vi "Teleop.vi"(10 "Match Info":T1={"Autonomous Elapsed Seconds"=0.0, "TeleOp Elapsed Seconds"=0.0, "Disabled Elapsed Seconds"=0.0, "Visited Autonomous"=FALSE, "Visited TeleOp"=FALSE, "Visited Disabled"=FALSE, "Autonomous Settings"={"Autonomous Style"=enum."Independent", "VI Refnum"=refnum}}, 11 "Call Context":T2) -> ()   [LabVIEW 2018]
doc: "This VI is called for each enabled TeleOp packet received from the DS. It is typically used to read from joysticks and other inputs and update I/O or setpoints for timed control loops. It should complete and return within 20 milliseconds or risk missing DS packets."
uses:
  <vilib>/Rock Robotics/WPI/DriverStation/WPI_DriverStationDerivedRobotMode.ctl
  <vilib>/Rock Robotics/WPI/DriverStation/WPI_DriverStationMatch Info.ctl
  <vilib>/Rock Robotics/WPI/Utilities/WPI_GetSetVariantRefNum.vi
  <vilib>/Rock Robotics/Network Tables/NT Write Boolean Array.vi
  <vilib>/Rock Robotics/Network Tables/NT Write Numeric Array.vi
  Global Variables/Yaw.vi
  <vilib>/Rock Robotics/WPI/RobotDrive/WPI_RobotDriveMecanumDrive_Cartesian.vi
  <vilib>/Rock Robotics/Network Tables/NT Write Boolean.vi
  <vilib>/Rock Robotics/Network Tables/NT Write Number.vi
  Global Variables/Strafe Correction TF.vi
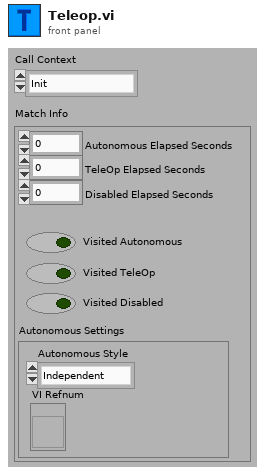
[diagram p1: front panel]
types:
  T1 = typedef "WPI_DriverStationMatch Info.ctl" = cluster{"Autonomous Elapsed Seconds":dbl, "TeleOp Elapsed Seconds":dbl, "Disabled Elapsed Seconds":dbl, "Visited Autonomous":bool, "Visited TeleOp":bool, "Visited Disabled":bool, "Autonomous Settings":cluster{"Autonomous Style":enum16{"Iterative", "Independent"}, "VI Refnum":refnum<vi>}}
  T2 = typedef "WPI_DriverStationDerivedRobotMode.ctl" = enum16{"Init", "Execute", "Stop"}
  T3 = typedef "WPI_SwitchDevRef.ctl" = cluster{"DevStatus":errorcluster, "DIO Channel":T4, "CntIndex":T5, "Normally Closed":bool}
  T4 = typedef "FPGA_DIOChannel.ctl" = enum8{"DIO 0", "DIO 1", "DIO 2", "DIO 3", "DIO 4", "DIO 5", "DIO 6", "DIO 7", "DIO 8", "DIO 9", "DIO MXP 0", "DIO MXP 1", "DIO MXP 2", "DIO MXP 3", "DIO MXP 4", "DIO MXP 5", "DIO MXP 6", "DIO MXP 7", "DIO MXP 8", "DIO MXP 9", "DIO MXP 10", "DIO MXP 11", "DIO MXP 12", "DIO MXP 13", "DIO MXP 14", "DIO MXP 15", "SPI Port CS1", "SPI Port CS2", "SPI Port CS3", "SPI Port MISO", "SPI Port MOSI", "Invalid"}
  T5 = typedef "FPGA_CounterCtrSystemIndex.ctl" = enum8{"Ctr 0", "Ctr 1", "Ctr 2", "Ctr 3", "Ctr 4", "Ctr 5", "Ctr 6", "Ctr 7", "Invalid"}
  T6 = typedef "WPI_JoystickDevRef.ctl" = cluster{"Device":T7}
  T7 = typedef "WPI_JoystickDeviceEnum.ctl" = enum16{"USB 0", "USB 1", "USB 2", "USB 3", "USB 4", "USB 5"}
  T8 = typedef "WPI_CompressorDevRef.ctl" = cluster{"DevStatus":errorcluster, "Pneumatics Control Module":u8}
  T9 = typedef "Command Status Info.ctl" = cluster{"Name":string, "Status":T10, "notifier out":T11}
  T10 = typedef "Completion Status.ctl" = enum16{"Successful", "Aborted", "Incomplete"}
  T11 = typedef "Completion Notifier.ctl" = refnum<notifier>
  T12 = typedef "WPI_RobotDriveDevRef.ctl" = cluster{"DevStatus":errorcluster, "Motors[]":T13[], "Square Inputs":bool, "Max Output":dbl}
  T13 = typedef "WPI_MotorControlDeviceRef.ctl" = cluster{"DeviceStatus":errorcluster, "Type":T14, "PWM":cluster{"PWM Channel":T15, "DeadBand":T16}, "CAN":cluster{"Device Number":u8, "SetOutput VI Ref":variant, "GetOutput VI Ref":variant, "Enable VI Ref":variant, "Disable VI Ref":variant, "Data":variant}, "Invert":bool, "DIO PWM":cluster{"PWM \"Enable\" Channel":T15, "DIOChannel":T4, "PWM Rate":dbl}}
  T14 = typedef "WPI_MotorControlType.ctl" = enum16{"PWM", "CAN", "DIO PWM"}
  T15 = typedef "FPGA_DIOPWMChannel.ctl" = enum8{"PWM 0", "PWM 1", "PWM 2", "PWM 3", "PWM 4", "PWM 5", "PWM 6", "PWM 7", "PWM 8", "PWM 9", "PWM MXP 0", "PWM MXP 1", "PWM MXP 2", "PWM MXP 3", "PWM MXP 4", "PWM MXP 5", "PWM MXP 6", "PWM MXP 7", "PWM MXP 8", "PWM MXP 9", "Invalid"}
  T16 = typedef "WPI_PWMDeadband.ctl" = cluster{"Name":string, "maxPositivePwm":i32, "minPositivePwm":i32, "centerPwm":i32, "maxNegativePwm":i32, "minNegativePwm":i32, "angularRange":u16}
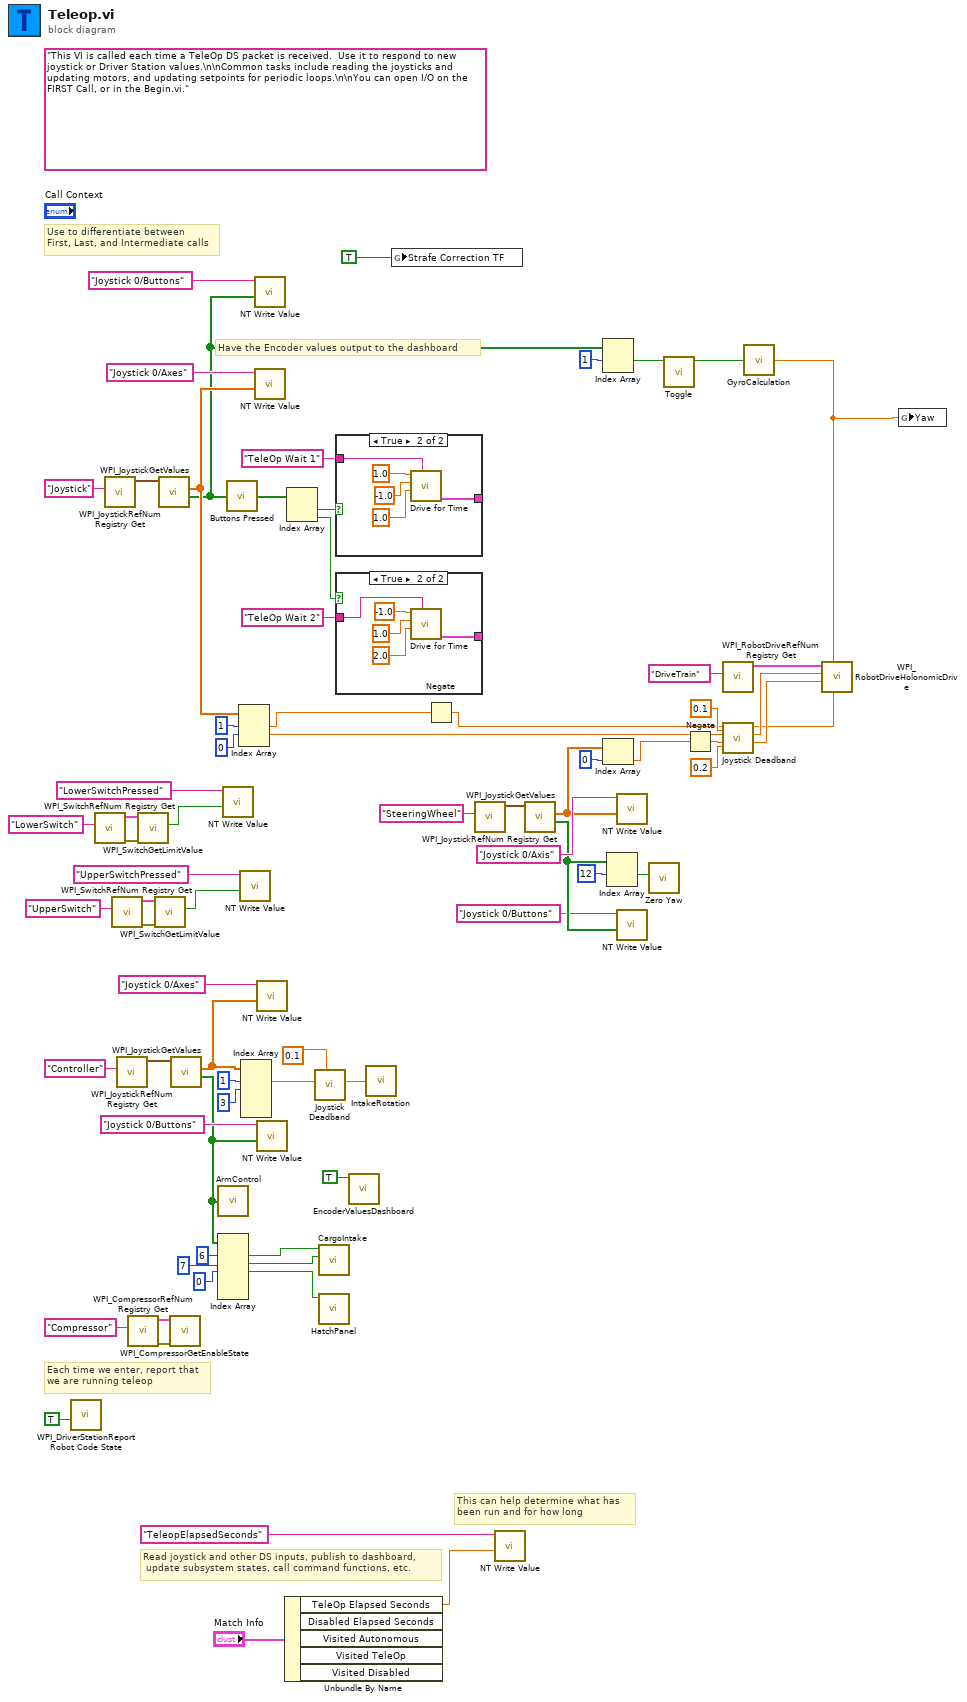
[diagram p0: block diagram]
diagram:
  (unwired) "This VI is called each time a TeleOp DS packet is received.  Use it to respond to new joystick or Driver Station values.\n\nCommon tasks include reading the joysticks and updating motors, and updating setpoints for periodic loops.\n\nYou can open I/O on the FIRST Call, or in the Begin.vi."
  # "Have the Encoder values output to the dashboard"
  # "Read joystick and other DS inputs, publish to dashboard,\n update subsystem states, call command functions, etc."
  # "Each time we enter, report that\nwe are running teleop"
  # "Use to differentiate between\nFirst, Last, and Intermediate calls"
  # "This can help determine what has\nbeen run and for how long"
  n1 = call <vilib>:"WPI_DriverStationReport Robot Code State.vi"("TeleOp"=TRUE ("Autonomous")) -> ()  [unwired: 10 in, 1 out]
  n2 = call <vilib>:"WPI_SwitchRefNum Registry Get.vi"("refnum name"="LowerSwitch") -> ("error out"=w31:errorcluster, "SwitchDevRef"=w30:T3)  [unwired: 9 in]
  n3 = call <vilib>:"WPI_JoystickRefNum Registry Get.vi"("refnum name"="Joystick") -> ("JoystickDevRef"=w71:T6)  [unwired: 1 in, 9 out]
  n4 = call <vilib>:"WPI_SwitchRefNum Registry Get.vi"("refnum name"="UpperSwitch") -> ("error out"=w26:errorcluster, "SwitchDevRef"=w25:T3)  [unwired: 9 in]
  n5 = call <vilib>:"WPI_JoystickRefNum Registry Get.vi"("refnum name"="Controller") -> ("JoystickDevRef"=w59:T6)  [unwired: 1 in, 9 out]
  n6 = call <vilib>:"WPI_CompressorRefNum Registry Get.vi"("refnum name"="Compressor") -> ("error out"=w39:errorcluster, "CompressorDevRef"=w38:T8)  [unwired: 9 in]
  n7 = call <vilib>:"WPI_SwitchGetLimitValue.vi"("error in (no error)"=w31, "SwitchDevRef"=w30) -> ("Switch Pressed"=w29:bool)  [unwired: 7 in, 2 out]
  n8 = call <vilib>:"WPI_SwitchGetLimitValue.vi"("error in (no error)"=w26, "SwitchDevRef"=w25) -> ("Switch Pressed"=w18:bool)  [unwired: 7 in, 2 out]
  n9 = call <vilib>:"WPI_JoystickGetValues.vi"("JoystickDevRef"=w71) -> ("Buttons"=w36:bool[], "Axes"=w64:dbl[])  [unwired: 6 in, 3 out]
  n10 = call <vilib>:"WPI_CompressorGetEnableState.vi"("error in (no error)"=w39, "CompressorDevRef"=w38) -> ()  [unwired: 6 in, 4 out]
  n11 = call <vilib>:"WPI_JoystickGetValues.vi"("JoystickDevRef"=w59) -> ("Buttons"=w14:bool[], "Axes"=w58:dbl[])  [unwired: 6 in, 3 out]
  n12 = call "ArmControl.vi"("ButtonArray"=w14) -> ()
  n13 = Index Array(array=w14, index #1=6 ("index"), index #2=7 ("index"), index #3=0 ("index")) -> (element #1=w12:bool, element #2=w13:bool, element #3=w9:bool)  [unwired: 3 in, 3 out]
  n14 = call-poly <vilib>:"NT Write Value.vi"("Boolean"=w29, "Name"="LowerSwitchPressed") -> ()  [unwired: 9 in, 1 out]
  n15 = call "Buttons Pressed.vi"("Button Values"=w36) -> ("Button Presses"=w68:bool[])
  n16 = Index Array(array=w64, index #1=1 ("index"), index #2=0 ("index")) -> (element #1=w17:dbl, element #2=w3:dbl)  [unwired: 1 in, 1 out]
  n17 = call-poly <vilib>:"NT Write Value.vi"("Boolean"=w18, "Name"="UpperSwitchPressed") -> ()  [unwired: 9 in, 1 out]
  n18 = Index Array(array=w58, index #1=1 ("index"), index #2=3 ("index")) -> (element #1=w15:dbl)  [unwired: 3 in, 4 out]
  n19 = call-poly <vilib>:"NT Write Value.vi"("Boolean Array"=w36, "Name"="Joystick 0/Buttons") -> ()  [unwired: 9 in, 1 out]
  n20 = call-poly <vilib>:"NT Write Value.vi"("Numeric Array"=w64, "Name"="Joystick 0/Axes") -> ()  [unwired: 9 in, 1 out]
  n21 = call-poly <vilib>:"NT Write Value.vi"("Numeric Array"=w58, "Name"="Joystick 0/Axes") -> ()  [unwired: 9 in, 1 out]
  n22 = call-poly <vilib>:"NT Write Value.vi"("Boolean Array"=w14, "Name"="Joystick 0/Buttons") -> ()  [unwired: 9 in, 1 out]
  n23 = Unbundle By Name("Match Info") -> ("TeleOp Elapsed Seconds"=w23:dbl)  [unwired: 4 out]
  n24 = Index Array(array=w68) -> (element #1=w67:bool, element #2=w66:bool)  [unwired: 2 in]
  n25 = call "Joystick Deadband.vi"("X Y Deadband"=0.1, "Y"=w15) -> ("Y Out"=w35:dbl)  [unwired: 7 in, 2 out]
  n26 = call "CargoIntake.vi"("Outside Case"=w12, "Inside Case"=w13) -> ()  [unwired: 9 in]
  n27 = call "HatchPanel.vi"("Boolean"=w9) -> ()  [unwired: 11 in]
  n28 = case shown="True" w67 {
    tunnel: [_ w78] -> _
    tunnel: "TeleOp Wait 1" ("Description") -> [_ w77]
    frame False {
    }
    frame True {
      n29 = call "Drive for Time.vi"("Description"=w77, "Seconds"=1.0, "Right Speed"=-1.0, "Left Speed"=1.0) -> ("Command Info Out"=w78:T9)  [unwired: 7 in]
    }
  }
  n30 = case shown="True" w66 {
    tunnel: [_ w82] -> _
    tunnel: "TeleOp Wait 2" ("Description") -> [_ w81]
    frame False {
    }
    frame True {
      n31 = call "Drive for Time.vi"("Description"=w81, "Seconds"=2.0, "Right Speed"=1.0, "Left Speed"=-1.0) -> ("Command Info Out"=w82:T9)  [unwired: 7 in]
    }
  }
  n32 = call "EncoderValuesDashboard.vi"("Teleop?"=TRUE) -> ()  [unwired: 3 in, 1 out]
  n33 = call "IntakeRotation.vi"("Input"=w35) -> ()
  n34 = global write "Strafe Correction TF.vi" "Strafe Correction TF"(TRUE) -> ()
  n35 = Negate(x=w17) -> (-x=w16:dbl)
  n36 = call <vilib>:"WPI_JoystickRefNum Registry Get.vi"("refnum name"="SteeringWheel") -> ("JoystickDevRef"=w61:T6)  [unwired: 1 in, 9 out]
  n37 = call-poly <vilib>:"NT Write Value.vi"("Numeric"=w23, "Name"="TeleopElapsedSeconds") -> ()  [unwired: 9 in, 1 out]
  n38 = call <vilib>:"WPI_JoystickGetValues.vi"("JoystickDevRef"=w61) -> ("Buttons"=w53:bool[], "Axes"=w54:dbl[])  [unwired: 6 in, 3 out]
  n39 = Index Array(array=w36, index #1=1 ("index")) -> (element #1=w34:bool)  [unwired: 1 in, 1 out]
  n40 = Index Array(array=w54, index=0) -> (element=w20:dbl)
  n41 = Index Array(array=w53, index #1=12 ("index")) -> (element #1=w37:bool)  [unwired: 1 in, 1 out]
  n42 = call-poly <vilib>:"NT Write Value.vi"("Numeric Array"=w54, "Name"="Joystick 0/Axis") -> ()  [unwired: 9 in, 1 out]
  n43 = call-poly <vilib>:"NT Write Value.vi"("Boolean Array"=w53, "Name"="Joystick 0/Buttons") -> ()  [unwired: 9 in, 1 out]
  n44 = call <vilib>:"Zero Yaw.vi"("Zero"=w37) -> ()  [unwired: 11 in]
  n45 = call "Toggle.vi"("Input"=w34) -> ("Output"=w33:bool)  [unwired: 9 in, 1 out]
  n46 = Negate(x=w20) -> (-x=w19:dbl)
  n47 = call <vilib>:"WPI_RobotDriveRefNum Registry Get.vi"("refnum name"="DriveTrain") -> ("RobotDriveDevRef"=w7:T12)  [unwired: 9 in, 1 out]
  n48 = call "Joystick Deadband.vi"("Z Deadband"=0.2, "X Y Deadband"=0.1, "Z"=w19, "Y"=w3, "X"=w16) -> ("Z Out"=w5:dbl, "Y Out"=w6:dbl, "X Out"=w4:dbl)  [unwired: 4 in]
  n49 = call "GyroCalculation.vi"("NavX Enable"=w33) -> ("Yaw"=w1:dbl)
  n50 = call-poly <vilib>:"WPI_RobotDriveHolonomicDrive.vi"("Rotation"=w4, "Gyro Angle"=w1, "Y"=w5, "X"=w6, "RobotDriveDevRef"=w7) -> ()  [unwired: 4 in, 3 out]
  n51 = global write "Yaw.vi" "Yaw"(w1) -> ()
